vi "Convert Steering Frame Velocity to Wheel Frame.vi"(8 "error in (no error)":errorcluster, 9 "steering frame velocity":dbl[](array[numeric]), 11 "wheel in":refnum<class "NI_Robotics_Wheel.lvclass">) -> (0 "error out":errorcluster, 1 "wheel frame velocity":dbl[](array[numeric]), 3 "wheel out":refnum<class "NI_Robotics_Wheel.lvclass">)   [LabVIEW 2017, in "NI_Robotics_Wheel.lvclass"]
uses:
  <vilib>/robotics/Steering/Wheel/NI_Robotics_Wheel.lvclass
  <vilib>/robotics/Steering/Wheel/NI_Robotics_Wheel.lvclass/NI_Robotics_Wheel.ctl
  <vilib>/Analysis/NI_AALBase.lvlib
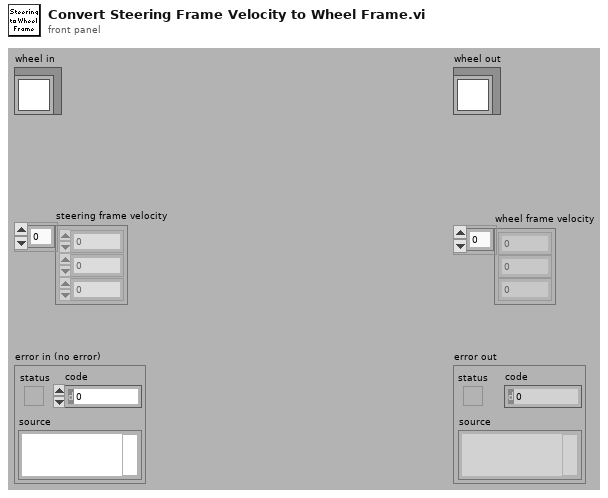
[diagram p1: front panel]
types:
  T1 = typedef "NI_Matrix.lvlib/RealMatrix.ctl" = dbl[][]
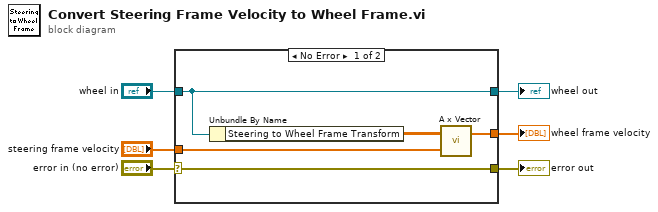
[diagram p0: block diagram]
diagram:
  n1 = case shown="No Error" "error in (no error)" {
    selector: "error in (no error)" -> [w9 w12]
    tunnel: "steering frame velocity" -> [w11 _]
    tunnel: [w10 _] -> w5
    tunnel: [w9 w12] -> w3
    tunnel: "wheel in" -> [w8 w13]
    tunnel: [w8 w13] -> w1
    frame No Error {
      n2 = Unbundle By Name(w8) -> ("Steering to Wheel Frame Transform"=w7:T1)
      n3 = call <vilib>:"A x Vector.vi"("Vector"=w11, "A"=w7) -> ("A x Vector"=w10:dbl[])  [unwired: 1 out]
    }
    frame Error {
    }
  }
  "error out" <- w3
  "wheel frame velocity" <- w5
  "wheel out" <- w1
